vi "Host - Get Slaves.vi"(8 "error in (no error)":errorcluster, 11 "Master Ref in":refnum<k21>) -> (0 "error out":errorcluster, 2 "Slaves":T1[](array[typedef]), 3 "Master Ref out":refnum<k21>)   [LabVIEW 2019, in "SEECD System Explorer.lvlib"]
uses:
  SEECD System Explorer.lvlib
  Type Defs/Host - Slave.ctl
  Type Defs/Host - Module.ctl
  <resource>/objmgr/IndComECAT.rc
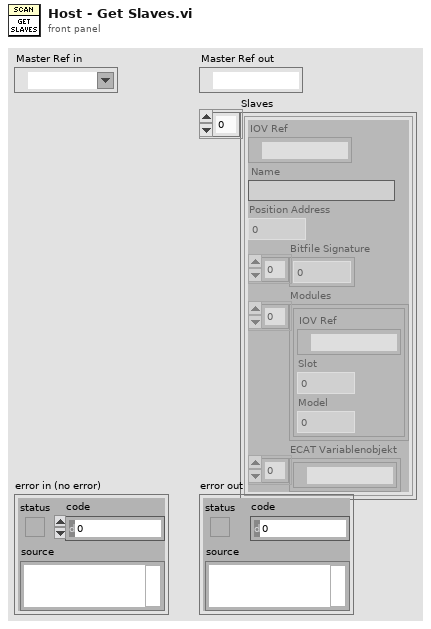
[diagram p1: front panel]
types:
  T1 = typedef "SEECD System Explorer.lvlib/Host - Slave.ctl" = cluster{"IOV Ref":refnum<k21>, "Name":string, "Position Address":u16, "Bitfile Signature":u8[], "Modules":T2[], "ECAT Variablenobjekt":refnum<k21>[]}
  T2 = typedef "SEECD System Explorer.lvlib/Host - Module.ctl" = cluster{"IOV Ref":refnum<k21>, "Slot":u32, "Model":u32}
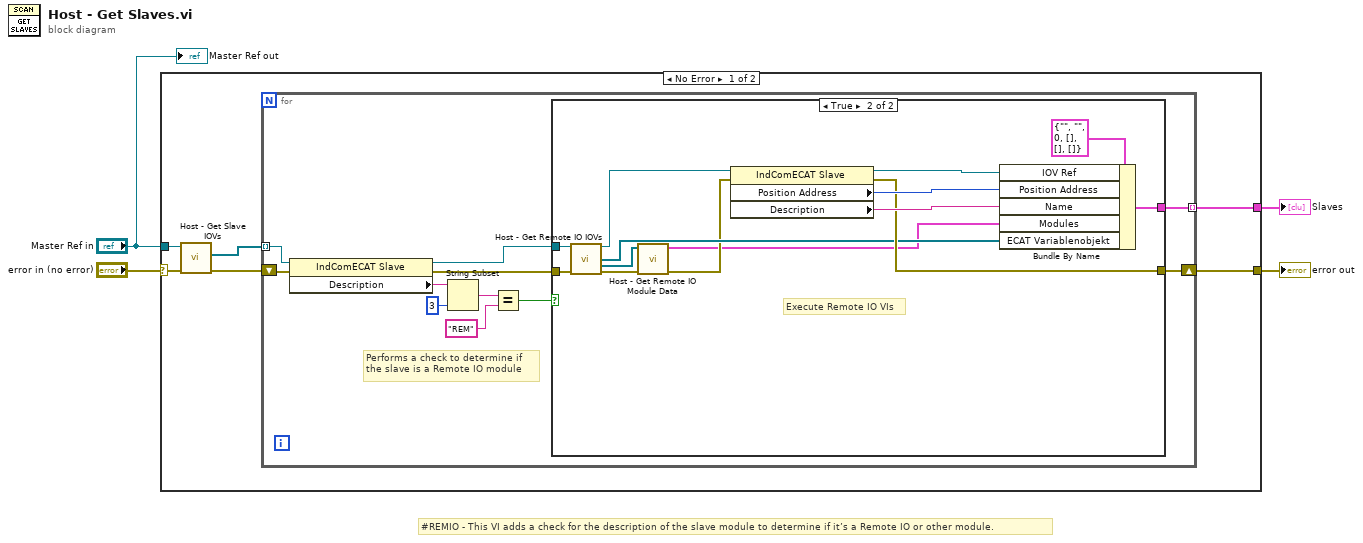
[diagram p0: block diagram]
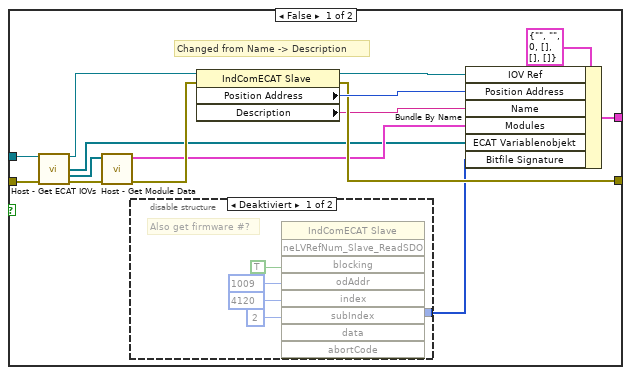
[diagram p2: hidden frame]
diagram:
  # "#REMIO - This VI adds a check for the description of the slave module to determine if it’s a Remote IO or other module."
  n1 = case shown="No Error" "error in (no error)" {
    selector: "error in (no error)" -> [w5 w56]
    tunnel: [w10 _] -> w4
    tunnel: [w9 w56] -> w3
    tunnel: "Master Ref in" -> [w8 _]
    frame No Error {
      n2 = call "Host - Get Slave IOVs.vi"("error in (no error)"=w5, "ECAT Master in"=w8) -> ("error IO"=w7:errorcluster, "All Slaves"=w6:refnum<k21>[])  [unwired: 7 in, 1 out]
      n3 = for {
        tunnel: w6 -> [w17] mode=indexing
        tunnel: [w20] -> w10 mode=indexing
        shift-right: [w19] -> w9
        shift-left: w7 -> [w21]
        # "Performs a check to determine if\nthe slave is a Remote IO module"
        n4 = property class="IndComECAT Slave"(reference=w17, error in=w21) -> (reference out=w16:refnum<k21>, error out=w18:errorcluster, "Description"=w15:string)
        n5 = String Subset(string=w15, length (rest)=3 ("length (rest)")) -> (substring=w13:string)  [unwired: 1 in]
        n6 = Equal?(x=w13, y="REM") -> (x = y?=w11:bool)
        n7 = case shown="True" w11 {
          tunnel: [w29 w50] -> w20
          tunnel: [w28 w51] -> w19
          tunnel: w18 -> [w23 w49]
          tunnel: w16 -> [w22 w48]
          frame False {
            # "Changed from Name -> Description"
            n8 = call "Host - Get ECAT IOVs.vi"("ECAT Slave in"=w22, "error in (no error)"=w23) -> ("ECAT Slave out"=w34:refnum<k21>, "ECAT Variablenobjekt"=w24:refnum<k21>[], "All Mods"=w36:refnum<k21>[], "error IO"=w35:errorcluster)  [unwired: 9 in, 1 out]
            n9 = call "Host - Get Module Data.vi"("error in (no error)"=w35, "Mod IOVs"=w36) -> ("error out"=w33:errorcluster, "Modules"=w26:T2[])  [unwired: 8 in]
            n10 = disable-structure shown="Deaktiviert" {
              disable-tunnel: [w37 _] -> w25
              frame Disabled {
                # "Also get firmware #?"
                n11 = invoke class="IndComECAT Slave" method="neLVRefNum_Slave_ReadSDO"("blocking"=TRUE, "odAddr"=u16 1009, "index"=u16 4120, "subIndex"=u8 2) -> ("data"=w37:u8[])  [unwired: 5 in, 8 out]
              }
              frame Enabled {
              }
            }
            n12 = property class="IndComECAT Slave"(reference=w34, error in=w33) -> (reference out=w31:refnum<k21>, error out=w28:errorcluster, "Position Address"=w30:u16, "Description"=w27:string)
            n13 = Bundle By Name(cluster=T1 {"IOV Ref"="", "Name"="", "Position Address"=0, "Bitfile Signature"=[], "Modules"=[], "ECAT Variablenobjekt"=[]} ("Slave"), "IOV Ref"=w31, "Position Address"=w30, "Name"=w27, "Modules"=w26, "ECAT Variablenobjekt"=w24, "Bitfile Signature"=w25) -> (w29:T1)
          }
          frame True {
            # "Execute Remote IO VIs"
            n14 = call "Host - Get Remote IO IOVs.vi"("ECAT Slave in"=w48, "error in (no error)"=w49) -> ("ECAT Slave out"=w47:refnum<k21>, "ECAT Variablenobjekt"=w46:refnum<k21>[], "All Remote IO Mods"=w42:refnum<k21>[], "error IO"=w45:errorcluster)  [unwired: 9 in, 1 out]
            n15 = call "Host - Get Remote IO Module Data.vi"("error in (no error)"=w45, "Remote IO Mod IOVs"=w42) -> ("error out"=w44:errorcluster, "Modules"=w43:T2[])  [unwired: 8 in]
            n16 = property class="IndComECAT Slave"(reference=w47, error in=w44) -> (reference out=w53:refnum<k21>, error out=w51:errorcluster, "Position Address"=w54:u16, "Description"=w55:string)
            n17 = Bundle By Name(cluster=T1 {"IOV Ref"="", "Name"="", "Position Address"=0, "Bitfile Signature"=[], "Modules"=[], "ECAT Variablenobjekt"=[]} ("Slave"), "IOV Ref"=w53, "Position Address"=w54, "Name"=w55, "Modules"=w43, "ECAT Variablenobjekt"=w46) -> (w50:T1)
          }
        }
      }
    }
    frame Error {
    }
  }
  "Slaves" <- w4
  "error out" <- w3
  "Master Ref out" <- "Master Ref in"
